vi "Logging Get Times.vi"(0 "Log Input":T1[](array[typedef])) -> (1 "Times":u32[](array[numeric]), 2 "Latest":u32)   [LabVIEW 2012, in "femtoRoboLib.lvlib"]
doc: "Takes a master log list (e.g. from Read All) and return a list of the timestamps that had at least one variable update, along with just the latest timestamp."
uses:
  femtoRoboLib.lvlib
  Controls/Log Entry - Full Block.ctl
  Controls/Log Entry.ctl
  Controls/Log Value Type.ctl
  Controls/Log Value Cluster.ctl
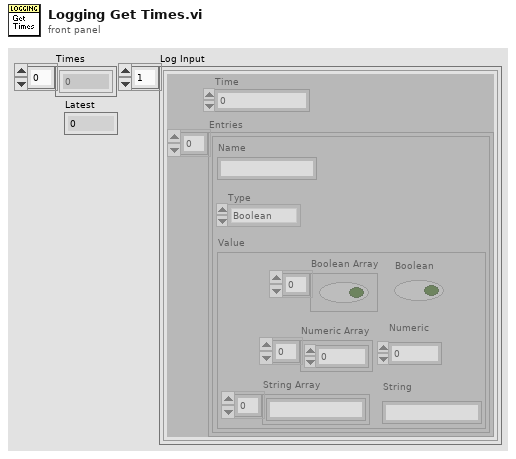
[diagram p1: front panel]
types:
  T1 = typedef "femtoRoboLib.lvlib/Log Entry - Full Block.ctl" = cluster{"Entries":T2[], "Time":u32}
  T2 = typedef "femtoRoboLib.lvlib/Log Entry.ctl" = cluster{"Name":string, "Type":T3, "Value":T4}
  T3 = typedef "femtoRoboLib.lvlib/Log Value Type.ctl" = enum16{"Boolean", "Numeric", "String", "Boolean Array", "Numeric Array", "String Array"}
  T4 = typedef "femtoRoboLib.lvlib/Log Value Cluster.ctl" = cluster{"Boolean Array":bool[], "Boolean":bool, "Numeric Array":dbl[], "Numeric":dbl, "String Array":string[], "String":string}
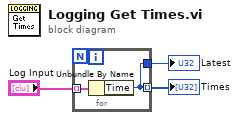
[diagram p0: block diagram]
diagram:
  n1 = for {
    tunnel: "Log Input" -> [w5] mode=indexing
    tunnel: [w4] -> w2 mode=indexing
    tunnel: [w4] -> w1
    n2 = Unbundle By Name(w5) -> ("Time"=w4:u32)
  }
  "Times" <- w2
  "Latest" <- w1
